vi "DPT Sort Data in Columns.vi"(0 "Q Element.Data":string[][](array[string]), 1 "DAQ Label List 2":string[](array[string]), 2 "Old Data Array":dbl[](array[numeric]), 3 "cDAQ Data Out":dbl[](array[numeric])) -> (7 "Output Data":string[][](array[string]), 8 "Array":string[](array[string]), 9 "New Data Array":dbl[](array[numeric]))   [LabVIEW 2016]
doc: "Stores measurements' label and data into 2D array."
panel:
  out "appended array 2":string[][](array[string])
  out "New label array":string[](array[string])
  out "New data array":string[](array[string])
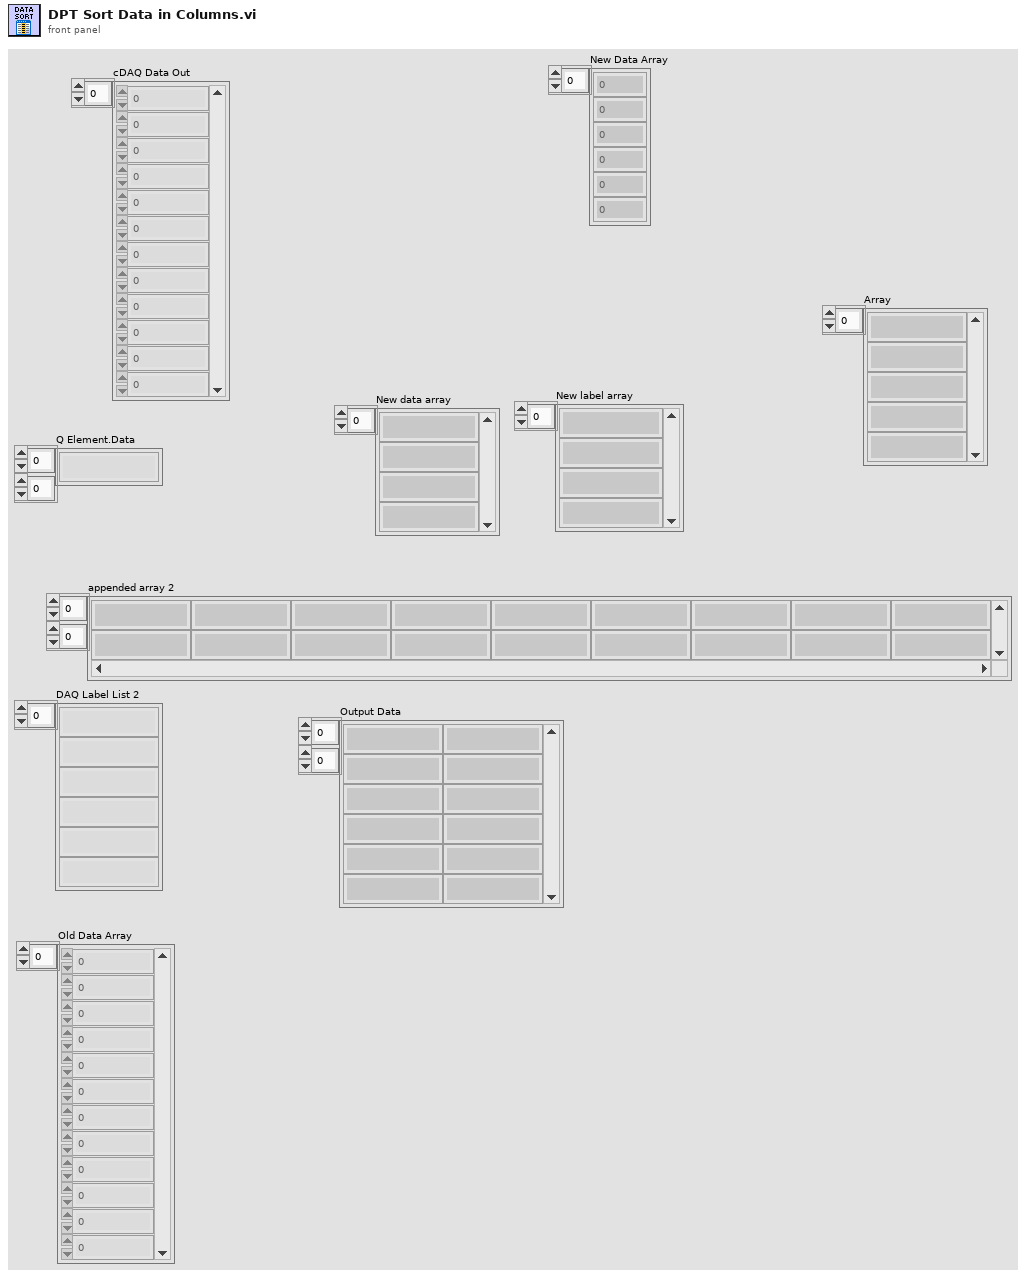
[diagram p1: front panel]
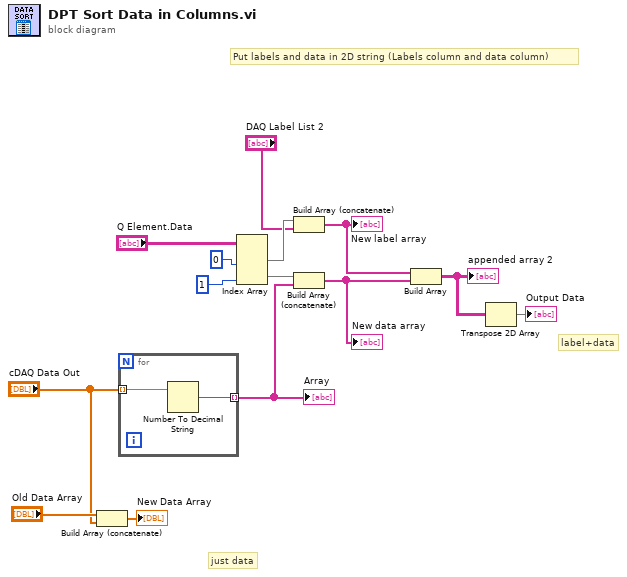
[diagram p0: block diagram]
diagram:
  # "label+data"
  # "just data"
  # "Put labels and data in 2D string (Labels column and data column)"
  n1 = Build Array (concatenate)("Old Data Array", "cDAQ Data Out") -> (→"New Data Array":dbl[])
  n2 = for {
    tunnel: [w16] -> w10 mode=indexing
    tunnel: "cDAQ Data Out" -> [w15] mode=indexing
    n3 = Number To Decimal String(number=w15) -> (decimal integer string=w16:string)  [unwired: 1 in]
  }
  "Array" <- w10
  n4 = Index Array(array="Q Element.Data", index (col) #1=0 ("disabled index (col)"), index (col) #2=1 ("index (col)")) -> (element #1=w13:string[], element #2=w11:string[])  [unwired: 2 in]
  n5 = Build Array (concatenate)(w13, "DAQ Label List 2") -> (w9:string[])
  "New label array" <- w9
  n6 = Build Array (concatenate)(w11, w10) -> (w8:string[])
  "New data array" <- w8
  n7 = Build Array(w9, w8) -> (w7:string[][])
  "appended array 2" <- w7
  n8 = Transpose 2D Array(2D array=w7) -> (transposed array=→"Output Data":string[][])
